vi "stillnessHelper (v00.00).vi"() -> ()   [LabVIEW 2022 SP3, in "stillnessHelper.lvclass"]
uses:
  stillnessHelper.lvclass
  stillnessHelper.lvclass/stillnessHelper.ctl
  stateMachine/statesWithOptions.ctl
panel:
  in  "Exit":bool
  in  "Task":enum32{"Task01", "appSettings"}(tab)
  out "appFolder":path
  in  "Application Name":string="stillnessHelper" caption="AppData sub-folder\nname - Write"
  out "States":string(combo)
  out "Options":string[](array[string])
  out "While Loop Index":i32
  out "error out":errorcluster
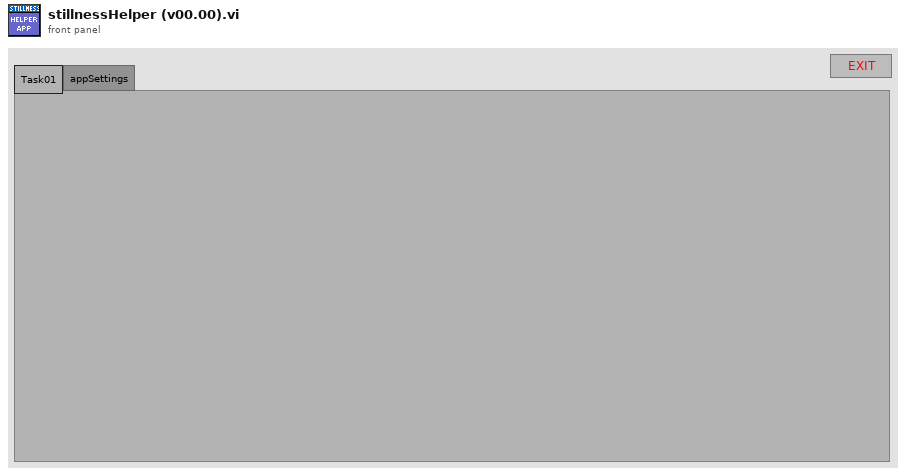
[diagram p1: front panel]
types:
  T1 = typedef "stillnessHelper.lvclass/statesWithOptions.ctl" = cluster{"States":string, "Options":string[]}
  T2 = enum32{"Invalid", "Standard", "Closed", "Hidden", "Minimized", "Maximized"}
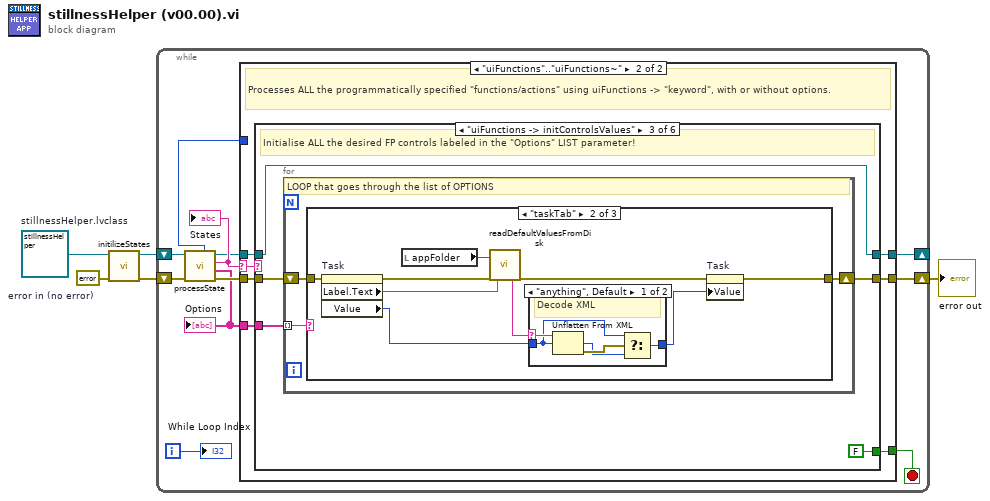
[diagram p0: block diagram]
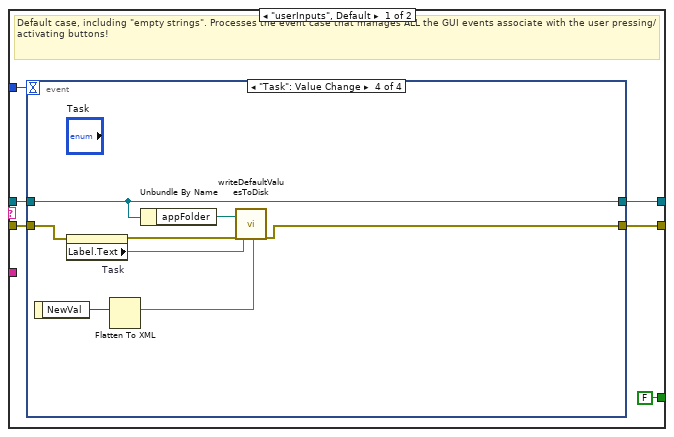
[diagram p2: hidden frame]
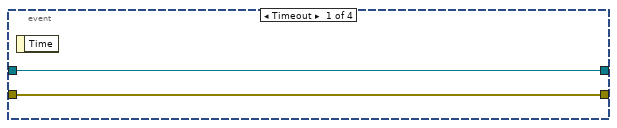
[diagram p3: hidden frame]
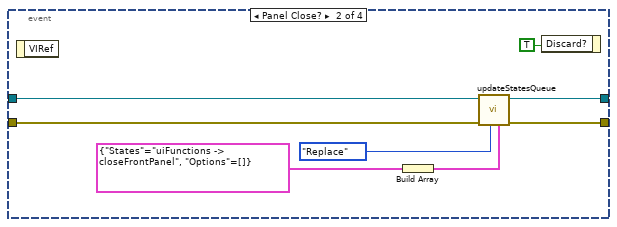
[diagram p4: hidden frame]
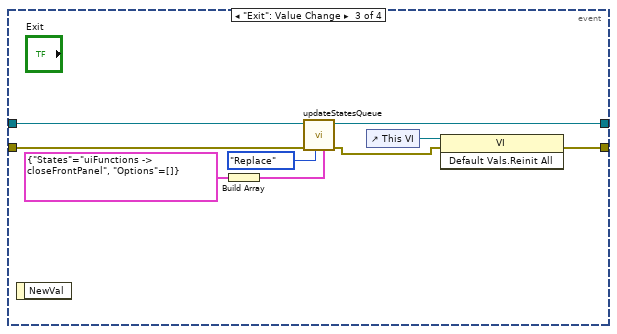
[diagram p5: hidden frame]
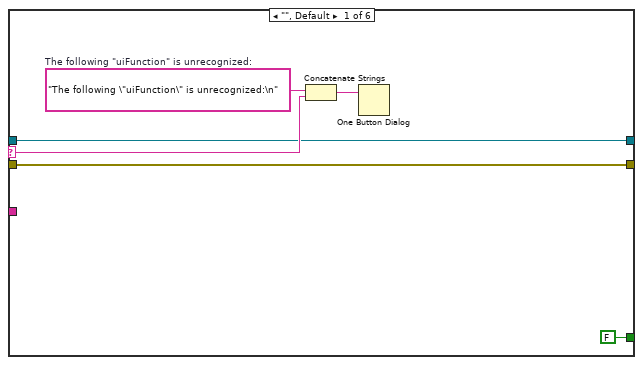
[diagram p6: hidden frame]
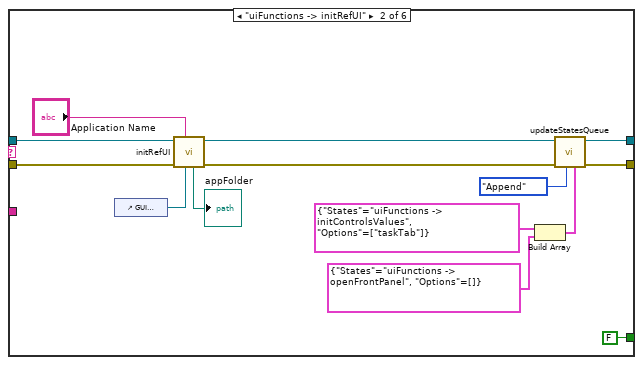
[diagram p7: hidden frame]
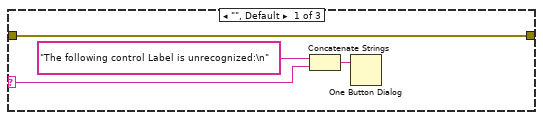
[diagram p8: hidden frame]
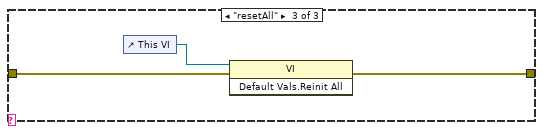
[diagram p10: hidden frame]
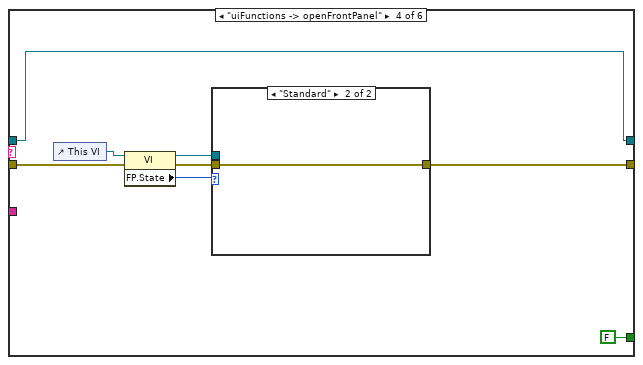
[diagram p11: hidden frame]
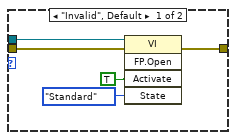
[diagram p12: hidden frame]
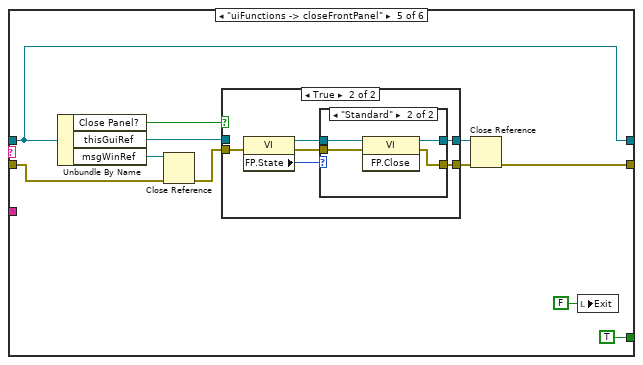
[diagram p13: hidden frame]
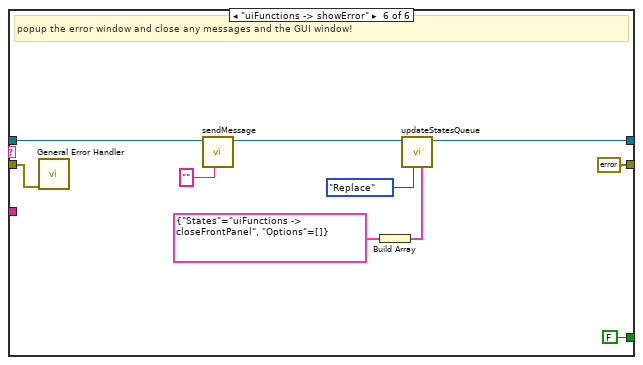
[diagram p16: hidden frame]
diagram:
  w3 = errorcluster {"status"=FALSE, "code"=0, "source"=""}  # error in (no error)
  w1 = refnum<class "stillnessHelper.lvclass"> refnum  # stillnessHelper.lvclass
  n1 = call "initilizeStates.vi"("error in (no error)"=w3, "guiTemplates in"=w1) -> ("error out"=w4:errorcluster, "guiTemplates out"=w5:refnum<class "stillnessHelper.lvclass">)  [unwired: 8 in]
  n2 = while {
    shift-right: [w12] -> w2
    shift-left: w4 -> [w15]
    shift-right: [w6] -> _
    shift-left: w5 -> [w16]
    i -> [w14]
    stop <- w8 stop-if-true
    n3 = call "processState.vi"("error in (no error)"=w15, "guiTemplates in"=w16) -> ("error out"=w11:errorcluster, "Options"=w7:string[], "States"=w13:string, "guiTemplates out"=w9:refnum<class "stillnessHelper.lvclass">, "Timeout"=w10:i32)  [unwired: 5 in]
    "Options" <- w7
    "States" <- w13
    n4 = case shown="\"uiFunctions\"..\"uiFunctions~\"" w13 {
      selector: w13 -> [_ w56]
      tunnel: [FALSE w55] -> w8
      tunnel: [w20 w54] -> w12
      tunnel: w11 -> [w19 w53]
      tunnel: w10 -> [w21 _]
      tunnel: w9 -> [w18 w52]
      tunnel: w7 -> [_ w51]
      tunnel: [w17 w50] -> w6
      frame "userInputs", Default {
        # "Default case, including \"empty strings\". Processes the event case that manages ALL the GUI events associate with the user pressing/activating buttons!"
        n5 = event shown="[3] \"Task\": Value Change" {
          selector: _ -> [_ _ _ _]
          dyn-events: _ -> [_ _ _ _]
          timeout: w21 -> [_ _ _ _]
          tunnel: [w24 w26 w33 w42] -> w20
          tunnel: w19 -> [w24 w29 w39 w48]
          tunnel: w18 -> [w23 w30 w40 w43]
          tunnel: [w23 w25 w36 w43] -> w17
          event Timeout {
            n6 = event-data() -> ()  [unwired: 1 in, 1 out]
          }
          event Panel Close? {
            n7 = event-data() -> ()  [unwired: 1 in, 1 out]
            n8 = Build Array(T1 {"States"="uiFunctions -> closeFrontPanel", "Options"=[]} ("States WITH Options")) -> (w27:T1[])
            n9 = call "updateStatesQueue.vi"("States Updates"=w27, "State Queue Options"=enum16{"Replace", "Append", "Prepend"}."Replace", "error in (no error)"=w29, "guiTemplates in"=w30) -> ("error out"=w26:errorcluster, "guiTemplates out"=w25:refnum<class "stillnessHelper.lvclass">)  [unwired: 6 in]
            n10 = event-data("Discard?"=TRUE) -> ()  [unwired: 1 in, 1 out]
          }
          event "Exit": Value Change {
            n11 = event-data() -> ()  [unwired: 1 in, 1 out]
            n12 = Build Array(T1 {"States"="uiFunctions -> closeFrontPanel", "Options"=[]} ("States WITH Options")) -> (w37:T1[])
            n13 = call "updateStatesQueue.vi"("States Updates"=w37, "State Queue Options"=enum16{"Replace", "Append", "Prepend"}."Replace", "error in (no error)"=w39, "guiTemplates in"=w40) -> ("error out"=w34:errorcluster, "guiTemplates out"=w36:refnum<class "stillnessHelper.lvclass">)  [unwired: 6 in]
            n14 = control-ref of="This VI"() -> (w35:refnum<vi>)
            n15 = invoke class="VI" method="Default Vals.Reinit All"(reference=w35, error in=w34) -> (error out=w33:errorcluster)  [unwired: 1 in, 2 out]
          }
          event "Task": Value Change {
            n16 = event-data() -> ("NewVal"=w49:enum32{"Task01", "appSettings"})  [unwired: 1 in]
            n17 = property on="Task" class="TabCtl (strict)"(error in=w48) -> (error out=w47:errorcluster, "Label.Text"=w45:string)  [unwired: 1 in, 1 out]
            n18 = Flatten To XML(6:w49) -> (2:w44:string)
            n19 = Unbundle By Name(w43) -> ("appFolder"=w46:path)
            n20 = call "writeDefaultValuesToDisk.vi"("appFolder"=w46, "error in (no error)"=w47, "Control Label"=w45, "Value (XML String)"=w44) -> ("error out"=w42:errorcluster)  [unwired: 15 in]
          }
        }
      }
      frame "uiFunctions".."uiFunctions~" {
        # "Processes ALL the programmatically specified \"functions/actions\" using uiFunctions -> \"keyword\", with or without options."
        n21 = case shown="\"uiFunctions -> initControlsValues\"" w56 {
          selector: w56 -> [w58 _ _ _ _ _]
          tunnel: [FALSE FALSE FALSE FALSE TRUE FALSE] -> w55
          tunnel: [w61 w76 w78 w110 w126 errorcluster {"status"=FALSE, "code"=0, "source"=""} ("error out")] -> w54
          tunnel: w53 -> [w61 w65 w79 w113 w124 w153]
          tunnel: w52 -> [w57 w70 w77 w107 w123 w152]
          tunnel: w51 -> [_ _ w80 _ _ _]
          tunnel: [w57 w63 w77 w107 w123 w149] -> w50
          frame "", Default {
            w60 = "The following \"uiFunction\" is unrecognized:\n"  # The following "uiFunction" is unrecognized:
            n22 = Concatenate Strings(w60, w58) -> (w59:string)
            n23 = One Button Dialog(message=w59) -> ()  [unwired: 1 in, 1 out]
          }
          frame "uiFunctions -> initRefUI" {
            n24 = control-ref of="GUI Reference"() -> (w67:refnum<vi>)
            n25 = call "initRefUI.vi"("main GUI Reference"=w67, "Application Name"="Application Name", "error in (no error)"=w65, "guiTemplates in"=w70) -> ("error out"=w64:errorcluster, "guiTemplates out"=w69:refnum<class "stillnessHelper.lvclass">, "App Folder"=→"appFolder":path)  [unwired: 5 in]
            n26 = Build Array(T1 {"States"="uiFunctions -> initControlsValues", "Options"=["taskTab"]} ("States WITH Options"), T1 {"States"="uiFunctions -> openFrontPanel", "Options"=[]} ("States WITH Options")) -> (w73:T1[])
            n27 = call "updateStatesQueue.vi"("States Updates"=w73, "State Queue Options"=enum16{"Replace", "Append", "Prepend"}."Append", "error in (no error)"=w64, "guiTemplates in"=w69) -> ("error out"=w76:errorcluster, "guiTemplates out"=w63:refnum<class "stillnessHelper.lvclass">)  [unwired: 6 in]
          }
          frame "uiFunctions -> initControlsValues" {
            # "Initialise ALL the desired FP controls labeled in the \"Options\" LIST parameter!"
            n28 = for {
              tunnel: w80 -> [w84] mode=indexing
              shift-right: [w83] -> w78
              shift-left: w79 -> [w82]
              # "LOOP that goes through the list of OPTIONS"
              n29 = case shown="\"taskTab\"" w84 {
                selector: w84 -> [w85 _ _]
                tunnel: [w88 w90 w105] -> w83
                tunnel: w82 -> [w88 w97 w106]
                frame "", Default {
                  n30 = Concatenate Strings("The following control Label is unrecognized:\n", w85) -> (w87:string)
                  n31 = One Button Dialog(message=w87) -> ()  [unwired: 1 in, 1 out]
                }
                frame "taskTab" {
                  n32 = property on="Task" class="TabCtl (strict)"(error in=w97) -> (error out=w96:errorcluster, "Label.Text"=w94:string, "Value"=w92:enum32{"Task01", "appSettings"})  [unwired: 1 in, 1 out]
                  n33 = local read "appFolder"() -> (w95:path)
                  n34 = call "readDefaultValuesFromDisk.vi"("appFolder"=w95, "error in (no error)"=w96, "Control Label"=w94) -> ("Value (XML String)"=w93:string, "error out"=w91:errorcluster)  [unwired: 14 in, 1 out]
                  n35 = case shown="\"anything\", Default" w93 {
                    selector: w93 -> [w102 _]
                    tunnel: [w98 w103] -> w89
                    tunnel: w92 -> [w100 w103]
                    frame "anything", Default {
                      # "Decode XML"
                      n36 = Unflatten From XML(xml string=w102, type=w100) -> (value=w99:enum32{"Task01", "appSettings"}, error out=w101:errorcluster)  [unwired: 1 in]
                      n37 = Select(t=w100, s=w101, f=w99) -> (s? t:f=w98:enum32{"Task01", "appSettings"})
                    }
                    frame "" {
                      # "NO File / Error"
                    }
                  }
                  n38 = property on="Task" class="TabCtl (strict)"(error in=w91, "Value"=w89) -> (error out=w90:errorcluster)  [unwired: 1 in, 1 out]
                }
                frame "resetAll" {
                  n39 = control-ref of="This VI"() -> (w104:refnum<vi>)
                  n40 = invoke class="VI" method="Default Vals.Reinit All"(reference=w104, error in=w106) -> (error out=w105:errorcluster)  [unwired: 1 in, 2 out]
                }
              }
            }
          }
          frame "uiFunctions -> openFrontPanel" {
            n41 = control-ref of="This VI"() -> (w112:refnum<vi>)
            n42 = property class="VI"(reference=w112, error in=w113) -> (reference out=w108:refnum<vi>, error out=w109:errorcluster, "FP.State"=w111:T2)
            n43 = case shown="\"Standard\"" w111 {
              tunnel: [w117 w120] -> w110
              tunnel: w109 -> [w119 w120]
              tunnel: w108 -> [w118 _]
              frame "Invalid", Default {
                n44 = invoke class="VI" method="FP.Open"(reference=w118, error in=w119, "Activate"=TRUE ("Activate?"), "State"=T2."Standard") -> (error out=w117:errorcluster)  [unwired: 1 in, 4 out]
              }
              frame "Standard" {
              }
            }
          }
          frame "uiFunctions -> closeFrontPanel" {
            n45 = Unbundle By Name(w123) -> ("Close Panel?"=w122:bool, "thisGuiRef"=w130:refnum<vi>, "msgWinRef"=w121:refnum<vi>)
            n46 = Close Reference(reference=w121, error in (no error)=w124) -> (error out=w129:errorcluster)
            n47 = case shown="True" w122 {
              tunnel: w130 -> [w132 _]
              tunnel: w129 -> [w133 w139]
              tunnel: [w132 w135] -> w128
              tunnel: [w133 w134] -> w127
              frame False {
              }
              frame True {
                n48 = property class="VI"(error in=w139) -> (reference out=w137:refnum<vi>, error out=w136:errorcluster, "FP.State"=w138:T2)  [unwired: 1 in]
                n49 = case shown="\"Standard\"" w138 {
                  tunnel: w137 -> [w141 w145]
                  tunnel: w136 -> [w140 w144]
                  tunnel: [w141 w143] -> w135
                  tunnel: [w140 w142] -> w134
                  frame "Invalid", Default {
                  }
                  frame "Standard" {
                    n50 = invoke class="VI" method="FP.Close"(reference=w145, error in=w144) -> (reference out=w143:refnum<vi>, error out=w142:errorcluster)  [unwired: 1 in, 1 out]
                  }
                }
              }
            }
            n51 = Close Reference(reference=w128, error in (no error)=w127) -> (error out=w126:errorcluster)
            n52 = local write "Exit"(FALSE ("Exit")) -> ()
          }
          frame "uiFunctions -> showError" {
            # "popup the error window and close any messages and the GUI window!"
            n53 = call <vilib>:"General Error Handler.vi"("error in (no error)"=w153) -> ()  [unwired: 10 in, 5 out]
            n54 = call "sendMessage.vi"("Message (\"\" => closes the window)"="" ("Message (\"\" => closes the window)"), "guiTemplates in"=w152) -> ("guiTemplates out"=w150:refnum<class "stillnessHelper.lvclass">)  [unwired: 8 in, 1 out]
            n55 = Build Array(T1 {"States"="uiFunctions -> closeFrontPanel", "Options"=[]} ("States WITH Options")) -> (w147:T1[])
            n56 = call "updateStatesQueue.vi"("States Updates"=w147, "State Queue Options"=enum16{"Replace", "Append", "Prepend"}."Replace", "guiTemplates in"=w150) -> ("guiTemplates out"=w149:refnum<class "stillnessHelper.lvclass">)  [unwired: 7 in, 1 out]
          }
        }
      }
    }
    "While Loop Index" <- w14
  }
  "error out" <- w2
